vi "GenerateUntriggeredStimulus.vi"(8 "error in (no error)":errorcluster, 11 "StimOnHeadBends in":refnum<class "StimOnHeadBends.lvclass">) -> (0 "error out":errorcluster, 2 "UntriggeredStimulusOut":sgl[][](array[numeric]), 3 "StimOnHeadBends out":refnum<class "StimOnHeadBends.lvclass">)   [LabVIEW 2019, in "StimOnHeadBends.lvclass"]
uses:
  StimOnHeadBends.lvclass
  StimOnHeadBends.lvclass/StimOnHeadBends.ctl
  ParametersGlobal.vi
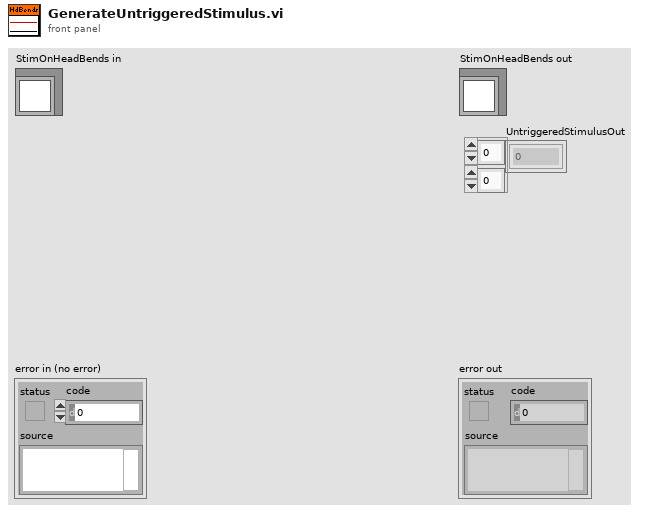
[diagram p1: front panel]
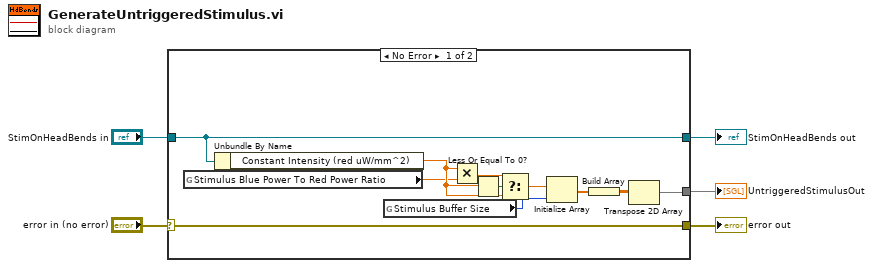
[diagram p0: block diagram]
diagram:
  n1 = case shown="No Error" "error in (no error)" {
    selector: "error in (no error)" -> [w16 w18]
    tunnel: [w16 w18] -> w2
    tunnel: [w15 w17] -> w4
    tunnel: "StimOnHeadBends in" -> [w15 w17]
    tunnel: [w6 _] -> w1
    frame No Error {
      n2 = global read "ParametersGlobal.vi" "Stimulus Blue Power To Red Power Ratio"() -> (w11:sgl)
      n3 = Unbundle By Name(w15) -> ("Constant Intensity (red uW/mm^2)"=w12:sgl)
      n4 = global read "ParametersGlobal.vi" "Stimulus Buffer Size"() -> (w9:i32)
      n5 = Multiply(x=w12, y=w11) -> (x*y=w14:sgl)
      n6 = Less Or Equal To 0?(x=w12) -> (x <= 0?=w13:bool)
      n7 = Select(t=w14, s=w13, f=w12) -> (s? t:f=w10:sgl)
      n8 = Initialize Array(w10, w9) -> (w8:sgl[])
      n9 = Build Array(w8) -> (w7:sgl[][])
      n10 = Transpose 2D Array(2D array=w7) -> (transposed array=w6:sgl[][])
    }
    frame Error {
    }
  }
  "error out" <- w2
  "StimOnHeadBends out" <- w4
  "UntriggeredStimulusOut" <- w1
